vi "1 port_Resistance Parameters_ksENA.vi"(0 "Port Measurements":T4, 2 "Specific Voltages 2":dbl[](array[numeric])=[32.0, 36.0], 5 "Selected Exp Settings":T1={"Floor_Sweep_Stop_V"=36.0, "Resistance Threshold"=1.0, "Floor_Sweep_Start_V"=36.0, "Floor_Sweep_Step_V"=1.0, "Roof_Sweep_Stop_V"=36.0, "Roof_Sweep_Start_V"=36.0, "Roof_Sweep_Step_V"=1.0, "Meas Type"=enum."Floor", "Experiment Name"=""}, 11 "Error In":errorcluster) -> (4 "Port Resistance Parametric Calculations":T3, 6 "Resistance Array Calc":T2, 15 "Error Out":errorcluster)   [LabVIEW 2013]
uses:
  Controls/Resistance Array Calculated Values.ctl
  Controls/Port Measurements.ctl
  Controls/Port Resistance Parametric Calculations.ctl
  Controls/Individual User Inputs_Floor and Roof.ctl
panel:
  out "Specific Voltages":dbl[](array[numeric])
  # "Test Settings"
  # "Calculation Settings"
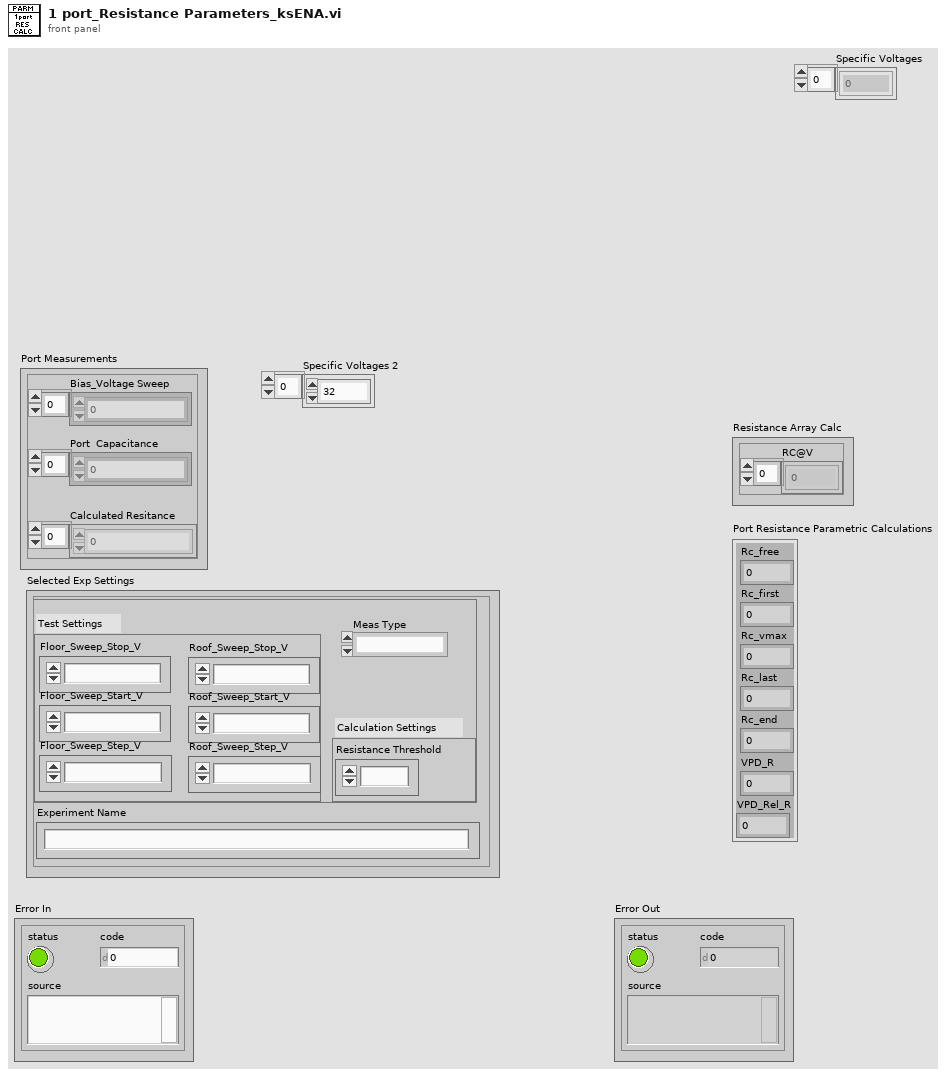
[diagram p1: front panel]
types:
  T1 = typedef "Individual User Inputs_Floor and Roof.ctl" = cluster{"Floor_Sweep_Stop_V":dbl, "Resistance Threshold":dbl, "Floor_Sweep_Start_V":dbl, "Floor_Sweep_Step_V":dbl, "Roof_Sweep_Stop_V":dbl, "Roof_Sweep_Start_V":dbl, "Roof_Sweep_Step_V":dbl, "Meas Type":enum16{"Floor", "Roof", "Floor and Roof"}, "Experiment Name":string}
  T2 = typedef "Resistance Array Calculated Values.ctl" = cluster{"RC@V":dbl[]}
  T3 = typedef "Port Resistance Parametric Calculations.ctl" = cluster{"Rc_free":dbl, "Rc_first":dbl, "Rc_vmax":dbl, "Rc_last":dbl, "Rc_end":dbl, "VPD_R":dbl, "VPD_Rel_R":dbl}
  T4 = typedef "Port Measurements.ctl" = cluster{"Bias_Voltage Sweep":dbl[], "Port  Capacitance":dbl[], "Calculated Resitance":dbl[]}
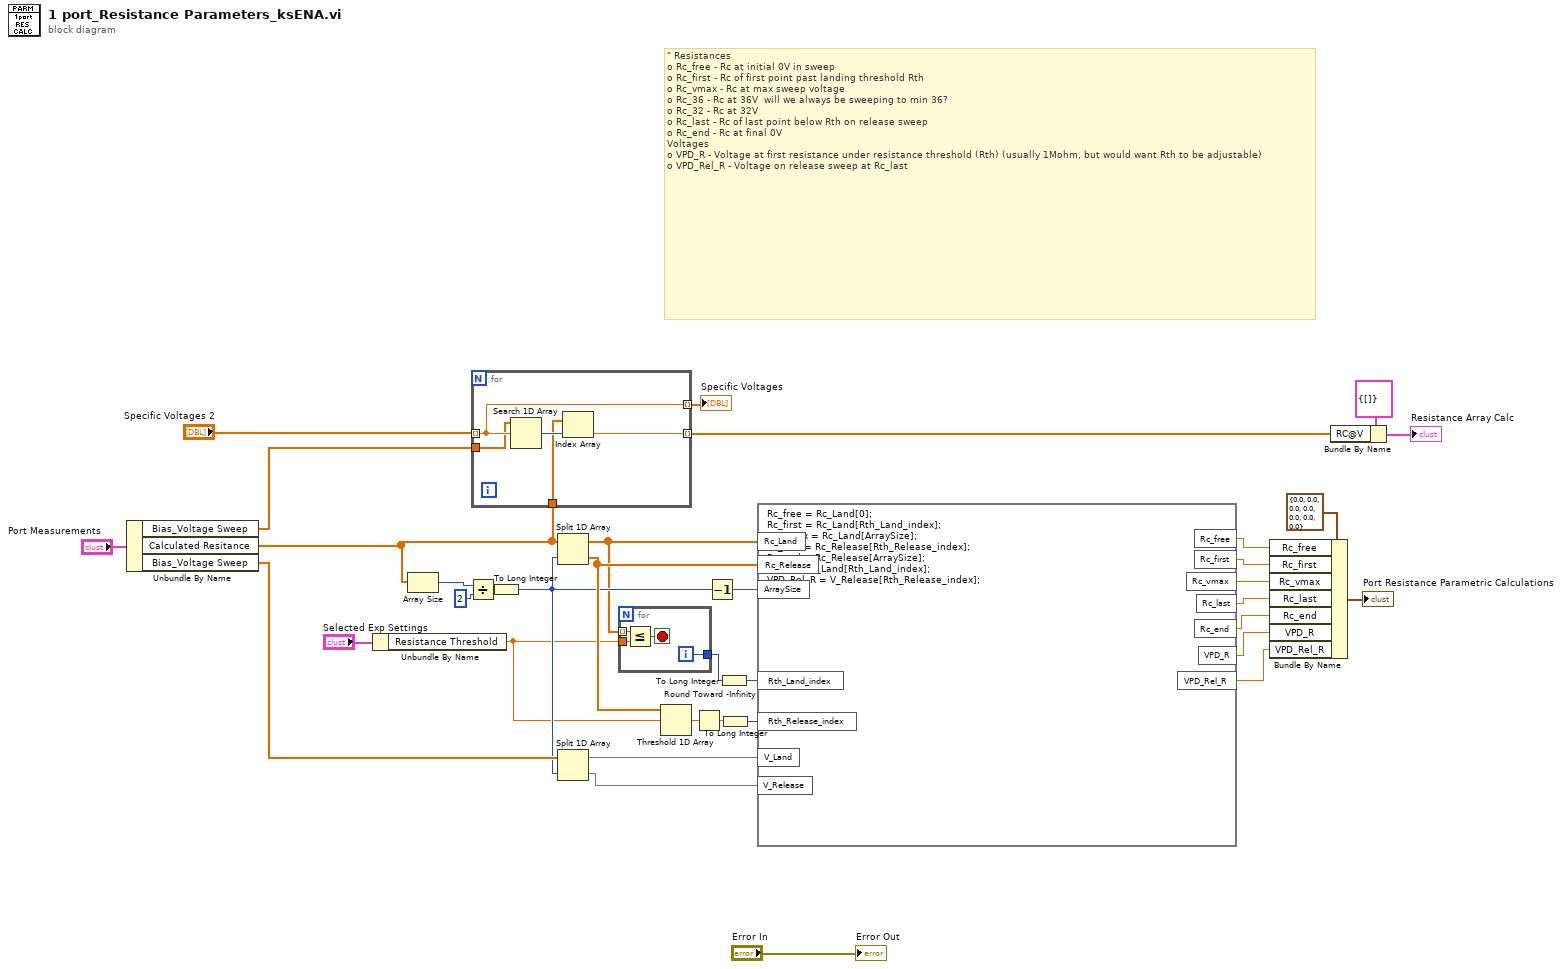
[diagram p0: block diagram]
diagram:
  # "\"\tResistances\no\tRc_free - Rc at initial 0V in sweep\no\tRc_first - Rc of first point past landing threshold Rth \no\tRc_vmax - Rc at max sweep voltage\no\tRc_36 - Rc at 36V  will we always be sweeping to min 36?\no\tRc_32 - Rc at 32V\no\tRc_last - Rc of last point below Rth on release sweep\no\tRc_end - Rc at final 0V\nVoltages\no\tVPD_R - Voltage at first resistance under resistance threshold (Rth) (usually 1Mohm, but would want Rth to be adjustable)\no\tVPD_Rel_R - Voltage on release sweep at Rc_last"
  n1 = Unbundle By Name("Port Measurements") -> ("Bias_Voltage Sweep"=w12:dbl[], "Calculated Resitance"=w6:dbl[], "Bias_Voltage Sweep"=w11:dbl[])
  n2 = Unbundle By Name("Selected Exp Settings") -> ("Resistance Threshold"=w1:dbl)
  n3 = Array Size(array=w6) -> (size(s)=w35:i32)
  n4 = Divide(x=w35, y=2) -> (x/y=w33:dbl)
  n5 = for {
    tunnel: "Specific Voltages 2" -> [w38] mode=indexing
    tunnel: [w39] -> w14 mode=indexing
    tunnel: [w38] -> w26 mode=indexing
    tunnel: w12 -> [w37]
    tunnel: w6 -> [w36]
    n6 = Search 1D Array(1D array=w37, element=w38) -> (index of element=w40:i32)  [unwired: 1 in]
    n7 = Index Array(array=w36, index=w40) -> (element=w39:dbl)
  }
  "Specific Voltages" <- w26
  n8 = To Long Integer(number=w33) -> (32bit integer=w10:i32)
  n9 = Split 1D Array(array=w6, index=w10) -> (first subarray=w8:dbl[], second subarray=w29:dbl[])
  n10 = Split 1D Array(array=w11, index=w10) -> (first subarray=w20:dbl[], second subarray=w19:dbl[])
  n11 = for {
    tunnel: [w44] -> w7
    tunnel: w8 -> [w43] mode=indexing
    tunnel: w1 -> [w42]
    i -> [w44]
    stop <- w41 stop-if-true
    n12 = Less Or Equal?(x=w43, y=w42) -> (x <= y?=w41:bool)
  }
  n13 = Threshold 1D Array(2:w1, 3:w29) -> (0:w31:dbl)  [unwired: 1 in]
  n14 = Round Toward -Infinity(1:w31) -> (0:w30:dbl)
  n15 = Decrement(x=w10) -> (x-1=w9:i32)
  n16 = To Long Integer(number=w7) -> (32bit integer=w32:i32)
  n17 = To Long Integer(number=w30) -> (32bit integer=w28:i32)
  n18 = formula code="Rc_free = Rc_Land[0];\nRc_first = Rc_Land[Rth_Land_index];\nRc_vmax = Rc_Land[ArraySize];\nRc_last = Rc_Release[Rth_Release_index];\nRc_end = Rc_Release[ArraySize];\nVPD_R = V_Land[Rth_Land_index];\nVPD_Rel_R = V_Release[Rth_Release_index];"("Rc_Land"=w8, "Rc_Release"=w29, "Rth_Land_index"=w32, "Rth_Release_index"=w28, "ArraySize"=w9, "V_Land"=w20, "V_Release"=w19) -> ("Rc_free"=w25:dbl, "Rc_first"=w24:dbl, "Rc_vmax"=w23:dbl, "Rc_last"=w22:dbl, "Rc_end"=w21:dbl, "VPD_R"=w18:dbl, "VPD_Rel_R"=w17:dbl)
  n19 = Bundle By Name(cluster=T3 {"Rc_free"=0.0, "Rc_first"=0.0, "Rc_vmax"=0.0, "Rc_last"=0.0, "Rc_end"=0.0, "VPD_R"=0.0, "VPD_Rel_R"=0.0} ("Port Resistance Parametric Calculations 2"), "Rc_free"=w25, "Rc_first"=w24, "Rc_vmax"=w23, "Rc_last"=w22, "Rc_end"=w21, "VPD_R"=w18, "VPD_Rel_R"=w17) -> (→"Port Resistance Parametric Calculations":T3)
  n20 = Bundle By Name(cluster=T2 {"RC@V"=[]} ("Resistance Array Calc"), "RC@V"=w14) -> (→"Resistance Array Calc":T2)
  "Error Out" <- "Error In"
